vi "PSO_UpdatePbestValues.vi"(6 "Parameters":T2={"Swarm size"=0, "Generations no."=0, "Cognitive coeff a1"=0.0, "Social coeff a2"=0.0, "Min inertia weight"=0.0, "Max inertia weight "=0.9, "Fmax"=0} {"Generations no." min=1; "Swarm size" min=1}, 11 "Population in":T1) -> (1 "GBest Fitness":dbl, 2 "Gbest Particle":i32[](array[numeric]), 3 "Population out":T1)   [LabVIEW 2016, in "Optimal Frequency Bands Search.lvlib" / "ParticleSwarm.lvlib"]
doc: "Обновить собственные лучшие значения координат для всех частиц"
uses:
  ParticleSwarm.lvlib
  PSO_tParameters.ctl
  PSO_tPopulation.ctl
panel:
  # "This VI is a part of BCI Design library, http://www.ru-bci.org \nCopyright © 2020, Sotnikov Peter, All rights reserved. License: CC BY-NC 4.0"
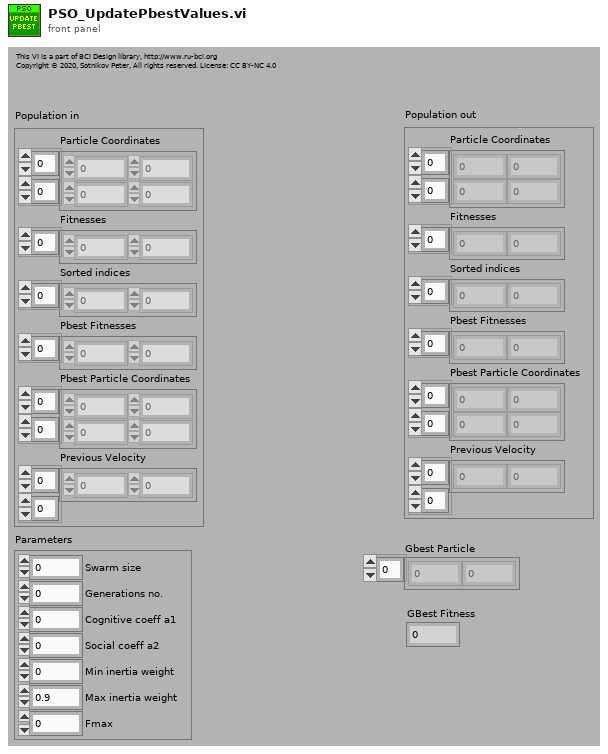
[diagram p1: front panel]
types:
  T1 = typedef "Optimal Frequency Bands Search.lvlib/ParticleSwarm.lvlib/PSO_tPopulation.ctl" = cluster{"Particle Coordinates":i32[][], "Fitnesses":dbl[], "Sorted indices":i32[], "Pbest Fitnesses":dbl[], "Pbest Particle Coordinates":i32[][], "Previous Velocity":dbl[][]}
  T2 = typedef "Optimal Frequency Bands Search.lvlib/ParticleSwarm.lvlib/PSO_tParameters.ctl" = cluster{"Swarm size":i32, "Generations no.":i32, "Cognitive coeff a1":dbl, "Social coeff a2":dbl, "Min inertia weight":dbl, "Max inertia weight ":dbl, "Fmax":i32}
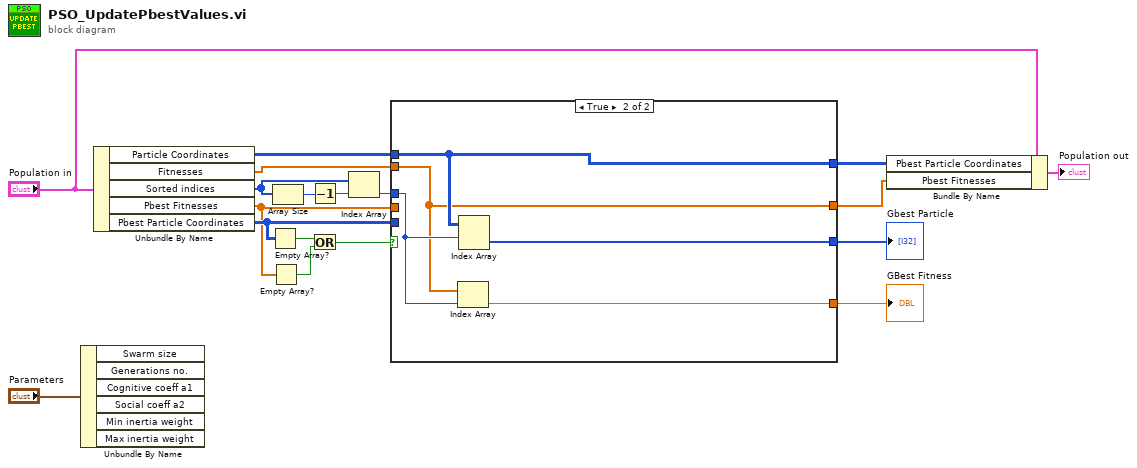
[diagram p0: block diagram]
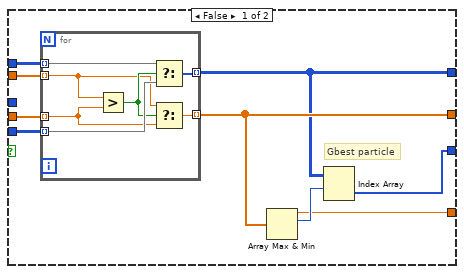
[diagram p2: hidden frame]
diagram:
  n1 = Unbundle By Name("Parameters") -> ()  [unwired: 6 out]
  n2 = Unbundle By Name("Population in") -> ("Particle Coordinates"=w4:i32[][], "Fitnesses"=w14:dbl[], "Sorted indices"=w17:i32[], "Pbest Fitnesses"=w12:dbl[], "Pbest Particle Coordinates"=w13:i32[][])
  n3 = Empty Array?(array=w13) -> (empty?=w11:bool)
  n4 = Empty Array?(array=w12) -> (empty?=w10:bool)
  n5 = Array Size(array=w17) -> (size(s)=w16:i32)
  n6 = Decrement(x=w16) -> (x-1=w15:i32)
  n7 = Or(x=w11, y=w10) -> (x .or. y?=w9:bool)
  n8 = Index Array(array=w17, index=w15) -> (element=w3:i32)
  n9 = case shown="True" w9 {
    tunnel: w14 -> [w27 w36]
    tunnel: w12 -> [w25 _]
    tunnel: w13 -> [w24 _]
    tunnel: [w20 w39] -> w7
    tunnel: [w21 w36] -> w6
    tunnel: w4 -> [w26 w39]
    tunnel: w3 -> [_ w37]
    tunnel: [w19 w38] -> w2
    tunnel: [w22 w35] -> w1
    frame False {
      # "Gbest particle"
      n10 = for {
        tunnel: w27 -> [w31] mode=indexing
        tunnel: w26 -> [w34] mode=indexing
        tunnel: w25 -> [w30] mode=indexing
        tunnel: w24 -> [w33] mode=indexing
        tunnel: [w29] -> w20 mode=indexing
        tunnel: [w28] -> w21 mode=indexing
        n11 = Greater?(x=w31, y=w30) -> (0:w32:bool)
        n12 = Select(t=w34, s=w32, f=w33) -> (s? t:f=w29:i32[])
        n13 = Select(t=w31, s=w32, f=w30) -> (s? t:f=w28:dbl)
      }
      n14 = Array Max & Min(array=w21) -> (max value=w22:dbl, max index (indices)=w23:i32)  [unwired: 2 out]
      n15 = Index Array(array=w20, index (row)=w23) -> (element=w19:i32[])  [unwired: 1 in]
    }
    frame True {
      n16 = Index Array(array=w36, index=w37) -> (element=w35:dbl)
      n17 = Index Array(array=w39, index (row)=w37) -> (element=w38:i32[])  [unwired: 1 in]
    }
  }
  "Gbest Particle" <- w2
  "GBest Fitness" <- w1
  n18 = Bundle By Name(cluster="Population in", "Pbest Particle Coordinates"=w7, "Pbest Fitnesses"=w6) -> (→"Population out":T1)
